vi "Falculator.vi"(1 "Op":string, 2 "Num2":dbl, 3 "Num1":dbl) -> (0 "Result":dbl)   [LabVIEW 2012]
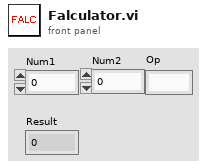
[diagram p1: front panel]
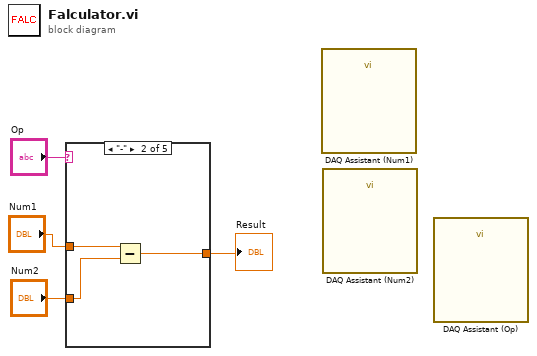
[diagram p0: block diagram]
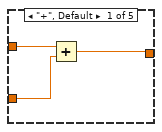
[diagram p2: hidden frame]
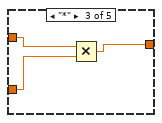
[diagram p3: hidden frame]
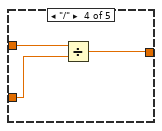
[diagram p4: hidden frame]
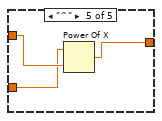
[diagram p5: hidden frame]
diagram:
  n1 = case shown="\"-\"" "Op" {
    tunnel: "Num1" -> [w7 w10 w13 w16 w18]
    tunnel: "Num2" -> [w6 w9 w12 w15 w17]
    tunnel: [w5 w8 w11 w14 w19] -> w1
    frame "+", Default {
      n2 = Add(x=w7, y=w6) -> (x+y=w5:dbl)
    }
    frame "-" {
      n3 = Subtract(x=w10, y=w9) -> (x-y=w8:dbl)
    }
    frame "*" {
      n4 = Multiply(x=w13, y=w12) -> (x*y=w11:dbl)
    }
    frame "/" {
      n5 = Divide(x=w16, y=w15) -> (x/y=w14:dbl)
    }
    frame "^" {
      n6 = Power Of X(1:w18, 2:w17) -> (0:w19:dbl)
    }
  }
  "Result" <- w1
  n7 = call "DAQ Assistant (Num1)"() -> ()  [unwired: 18 in, 2 out]
  n8 = call "DAQ Assistant (Num2)"() -> ()  [unwired: 18 in, 2 out]
  n9 = call "DAQ Assistant (Op)"() -> ()  [unwired: 18 in, 2 out]
